vi "JogZ.vi"(8 "error in":errorcluster, 9 "connection refnum in":refnum<k5>, 10 "Speed (units/s)":dbl min=0.0 max=1500.0, 11 "Units":enum16{"mm", "µm"}(ring)) -> (0 "error out":errorcluster, 1 "connection refnum out z":refnum<k5>)   [LabVIEW 2023]
doc: "Move in the Z direction until commanded to stop"
uses:
  GlobalVarsNetwork.vi
panel:
  in  "Stop Button":bool
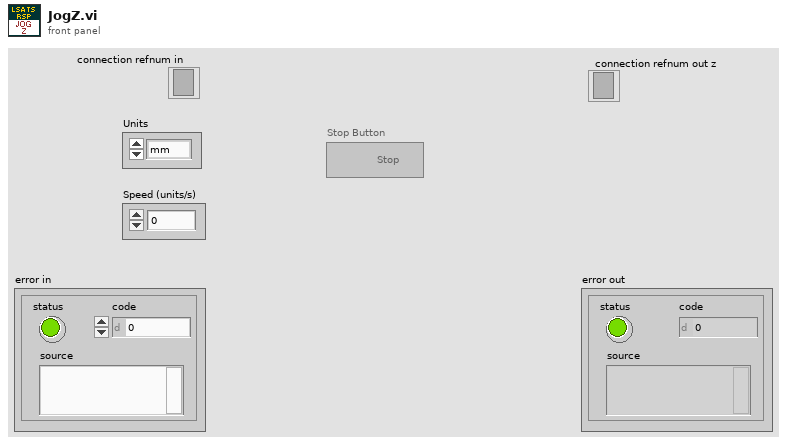
[diagram p1: front panel]
types:
  T1 = cluster{"XY_IP_ADDRESS":string, "Z_IP_ADDRESS":string, "Port":u16, "connection refnum x,y":refnum<k5>, "connection refnum z":refnum<k5>}
  T2 = enum8{"Enabled", "Disabled", "Disabled and Grayed Out"}
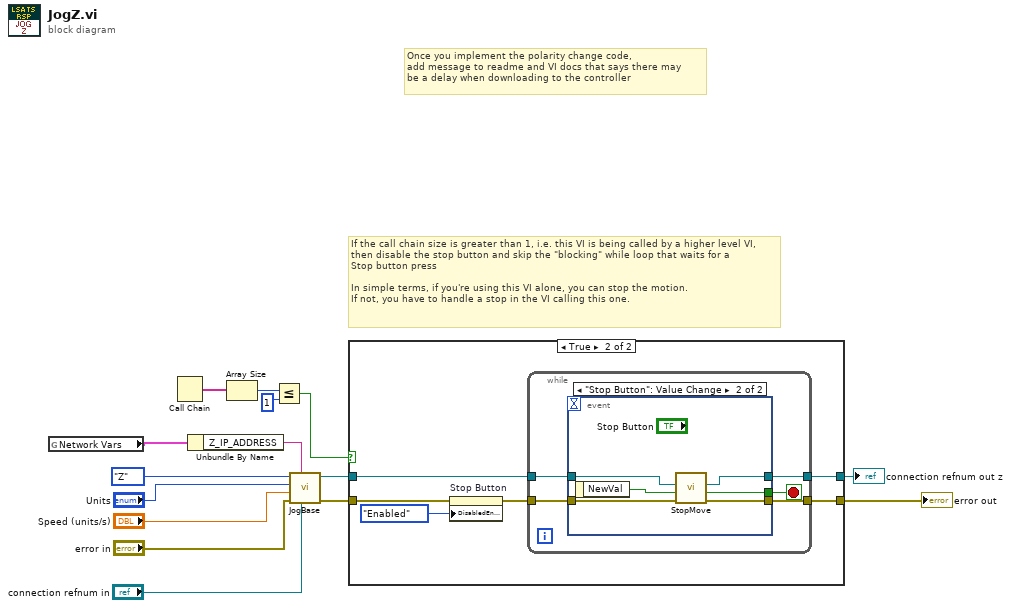
[diagram p0: block diagram]
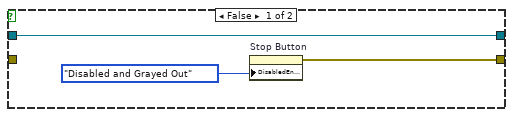
[diagram p2: hidden frame]
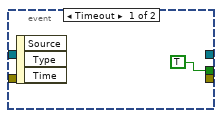
[diagram p3: hidden frame]
diagram:
  # "Once you implement the polarity change code,\nadd message to readme and VI docs that says there may \nbe a delay when downloading to the controller"
  # "If the call chain size is greater than 1, i.e. this VI is being called by a higher level VI,\nthen disable the stop button and skip the \"blocking\" while loop that waits for a \nStop button press\n\nIn simple terms, if you're using this VI alone, you can stop the motion.\nIf not, you have to handle a stop in the VI calling this one."
  n1 = global read "GlobalVarsNetwork.vi" "Network Vars"() -> (w10:T1)
  n2 = Call Chain() -> (call chain=w7:string[])
  n3 = Unbundle By Name(w10) -> ("Z_IP_ADDRESS"=w11:string)
  n4 = Array Size(array=w7) -> (size(s)=w5:i32)
  n5 = Less Or Equal?(x=w5, y=1) -> (x <= y?=w4:bool)
  n6 = call "JogBase.vi"("connection refnum in"="connection refnum in", "IP Address"=w11, "error in"="error in", "Speed"="Speed (units/s)", "Units"="Units", "Axis"=enum16{"Z", "Y", "X"}."Z") -> ("error out"=w9:errorcluster, "connection refnum out"=w2:refnum<k5>)  [unwired: 2 in]
  n7 = case shown="True" w4 {
    tunnel: [w18 w24] -> w8
    tunnel: w9 -> [_ w21]
    tunnel: w2 -> [w16 w20]
    tunnel: [w16 w19] -> w1
    frame False {
      n8 = property on="Stop Button" class="Bool"("DisabledEnum"=T2."Disabled and Grayed Out" ("Disabled")) -> (error out=w18:errorcluster)  [unwired: 2 in, 1 out]
    }
    frame True {
      n9 = property on="Stop Button" class="Bool"(error in=w21, "DisabledEnum"=T2."Enabled" ("Disabled")) -> (error out=w23:errorcluster)  [unwired: 1 in, 1 out]
      n10 = while {
        tunnel: w23 -> [w29]
        tunnel: [w28] -> w24
        tunnel: w20 -> [w26]
        tunnel: [w25] -> w19
        stop <- w27 stop-if-true
        n11 = event shown="[1] \"Stop Button\": Value Change" {
          selector: _ -> [_ _]
          dyn-events: _ -> [_ _]
          timeout: _ -> [_ _]
          tunnel: w29 -> [_ w36]
          tunnel: [_ w35] -> w28
          tunnel: [TRUE w34] -> w27
          tunnel: w26 -> [_ w32]
          tunnel: [_ w31] -> w25
          event Timeout {
            n12 = event-data() -> ()  [unwired: 1 in, 3 out]
          }
          event "Stop Button": Value Change {
            n13 = event-data() -> ("NewVal"=w33:bool)  [unwired: 1 in]
            n14 = call "StopMove.vi"("error in"=w36, "Stop?"=w33, "connection refnum in,  z"=w32) -> ("error out"=w35:errorcluster, "Stop?"=w34:bool, "connection refnum out z"=w31:refnum<k5>)  [unwired: 1 in, 1 out]
          }
        }
      }
    }
  }
  "error out" <- w8
  "connection refnum out z" <- w1
